vi "Msg To.vi"(9 "Insert (T) or Remove (F)":bool, 10 "Queue Nested":map{string, refnum<data-value>}(c390)) -> (3 "Update Queue Nested Msg Strategy out":refnum<class "Update Queue Nested Msg Strategy.lvclass">)   [LabVIEW 2021, in "jettl.lvlib" / "Update Queue Nested.lvlib" / "Update Queue Nested Msg Strategy.lvclass"]
uses:
  Update Queue Nested Msg Strategy.lvclass
  Msg Strategy/Msg Strategy.lvclass
  Update Queue Nested Msg Strategy.lvclass/Update Queue Nested Msg Strategy.ctl
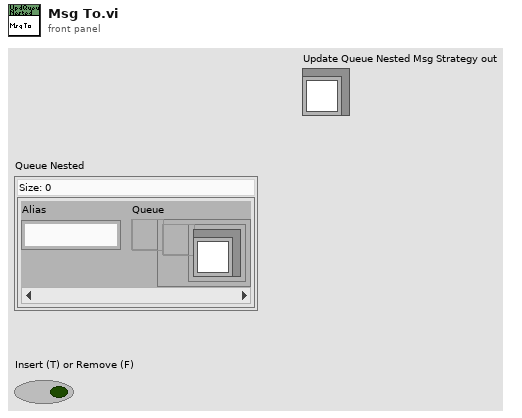
[diagram p1: front panel]
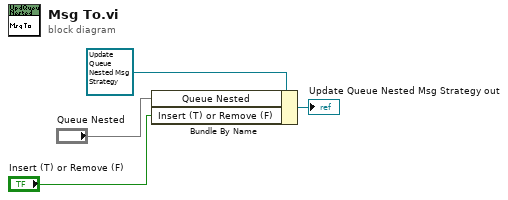
[diagram p0: block diagram]
diagram:
  n1 = Bundle By Name(cluster=refnum<class "Update Queue Nested Msg Strategy.lvclass"> refnum ("Update Queue Nested Msg out"), "Queue Nested"="Queue Nested", "Insert (T) or Remove (F)"="Insert (T) or Remove (F)") -> (→"Update Queue Nested Msg Strategy out":refnum<class "Update Queue Nested Msg Strategy.lvclass">)
